vi "Starter Kit 2.0 Custom RT Host Default.vi"() -> ()   [LabVIEW 2011]
doc: "This VI shows how to use hardware abstracted sensor drivers with a custom FPGA VI to control a Starter Kit robot. This VI runs on the RT host. The main FPGA VI must be compiled before this host VI can be run."
uses:
  <vilib>/userDefined/High Color/nirio_resource_hc.ctl
  <vilib>/Platform/TimedLoop/XDataNode/timing_clust.ctl
  <vilib>/Platform/TimedLoop/XDataNode/nitl_modes.ctl
  <vilib>/Platform/TimedLoop/XDataNode/wakeup.ctl
  <instrlib>/DC Motor Controller/HAIOL/DC Motor Controller.lvclass
  <instrlib>/Hitec HS400 Series/HAIOL/Hitec HS400 Series.lvclass
  <instrlib>/Parallax PING)))/HAIOL/Parallax PING))).lvclass
  <vilib>/robotics/Utilities/RPM to Radians per Second (Scalar).vi
  <vilib>/robotics/Utilities/Radians per Second to RPM (Scalar).vi
  <vilib>/FPGAPlugInAG/sbRIO-9632/niLvFpga_Open_sbRIO-9632.vi
  <vilib>/rvi/interface/common/dynamic/niFpgaDynamicAddResources.vi
  <vilib>/Utility/AngleManip/Degrees to Radians (Scalar DBL).vi
  <vilib>/Utility/error.llb/Error Cluster From Error Code.vi
  <vilib>/rvi/errors/niLvFpgaAdjustHostInterfaceError.vi
  <vilib>/FPGAPlugInAG/Dynamic/niLvFpga_Close_Dynamic.vi
  <vilib>/Platform/TimedLoop/XDataNode/XDataNode.xnode
  <vilib>/rvi/interface/nirviOpenFPGA/nirviOpenFPGA.xnode
  FPGA Bitfiles/MintaDaNIrobotho_FPGATarget_StarterKit2.0Cus_A15A34EB.lvbitx
  Starter Kit 2.0 Custom FPGA Main.vi
  <vilib>/rvi/interface/nirviReadWriteControl/nirviReadWriteControl.xnode
  <vilib>/rvi/interface/nirviCloseFPGA/nirviCloseFPGA.xnode
  <instrlib>/DC Motor Controller/HAIOL/FPGA/DC Motor Controller FPGA.lvclass
  <instrlib>/Hitec HS400 Series/HAIOL/FPGA/Hitec HS400 Series FPGA.lvclass
  <instrlib>/Parallax PING)))/HAIOL/FPGA/Parallax PING))) FPGA.lvclass
  <vilib>/robotics/Utilities/NI_Robotics Utilities.lvlib
  <vilib>/Utility/AngleManip/NI_AngleManipulation.lvlib
  <vilib>/rvi/interface/Simulation/niFpgaSimulationCallBeginRW.vi
  NiFpgaLv.dll
  <vilib>/Platform/TimedLoop/XDataNode/XDNodeRunTimeDep.lvlib
panel:
  out "CMPS03 angle":sgl(knob) scale=0.0..360.0 scale format="%#_4f"
  in  "stop":bool
  in  "Left":dbl(slide) min=-100.0 max=100.0 step=4.0 scale=-100.0..100.0
  in  "Right":dbl(slide) min=-100.0 max=100.0 step=4.0 scale=-100.0..100.0
  out "ccw motor velocities":cluster{"Left":dbl, dbl, "Right":dbl, dbl}(graph)
  in  "sensor motor angle":dbl(slide) caption="Sensor Motor Angle (degrees)" scale=90.0..-90.0
  out "PING))) Sensor Distance (m)":dbl(graph)
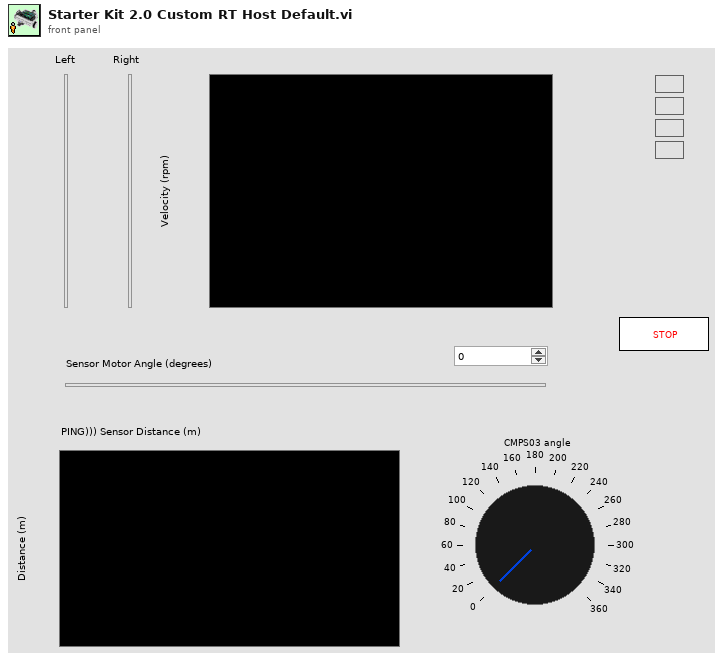
[diagram p1: front panel]
types:
  T1 = typedef "nirio_resource_hc.ctl" = tag
  T2 = typedef "XDNodeRunTimeDep.lvlib/timing_clust.ctl" = cluster{"Expected End [f-1]":u64, "Actual End [f-1]":u64, "Finished Late? [f-1]":bool, "Expected End [i-1]":u64, "Actual End [i-1]":u64, "Finished Late? [i-1]":bool, "Expected Start [i]":u64, "Actual Start [i]":u64, "Expected Start [f]":u64, "Actual Start [f]":u64, "Source Name":string, "Structure Name":string, "Period":i64, "Deadline":i64, "Offset":i64, "Start":i64, "Priority":i32, "Timeout":i32, "Mode":T3, "Wakeup Reason":T4, "Error":errorcluster, "Source Type":string, "Secondary Source Type":string, "Global End Time":u64, "Global Start Time":u64, "Frame Duration":u64, "Iteration Duration":u64, "Assigned CPU":i32, "I/O Scan Engine Mode":u32}
  T3 = typedef "XDNodeRunTimeDep.lvlib/nitl_modes.ctl" = enum32{"No Change", "Process missed periods, maintain original phase", "Discard missed periods, maintain original phase", "Process missed periods, ignore original phase", "Discard missed periods, ignore original phase"}
  T4 = typedef "XDNodeRunTimeDep.lvlib/wakeup.ctl" = enum32{"Normal", "Aborted", "Asynchronous wakeup", "Timing source error", "Timed loop error", "Timeout"}
  T5 = cluster{"Left":dbl, "rpm":dbl, "Right":dbl, "rpm":dbl}
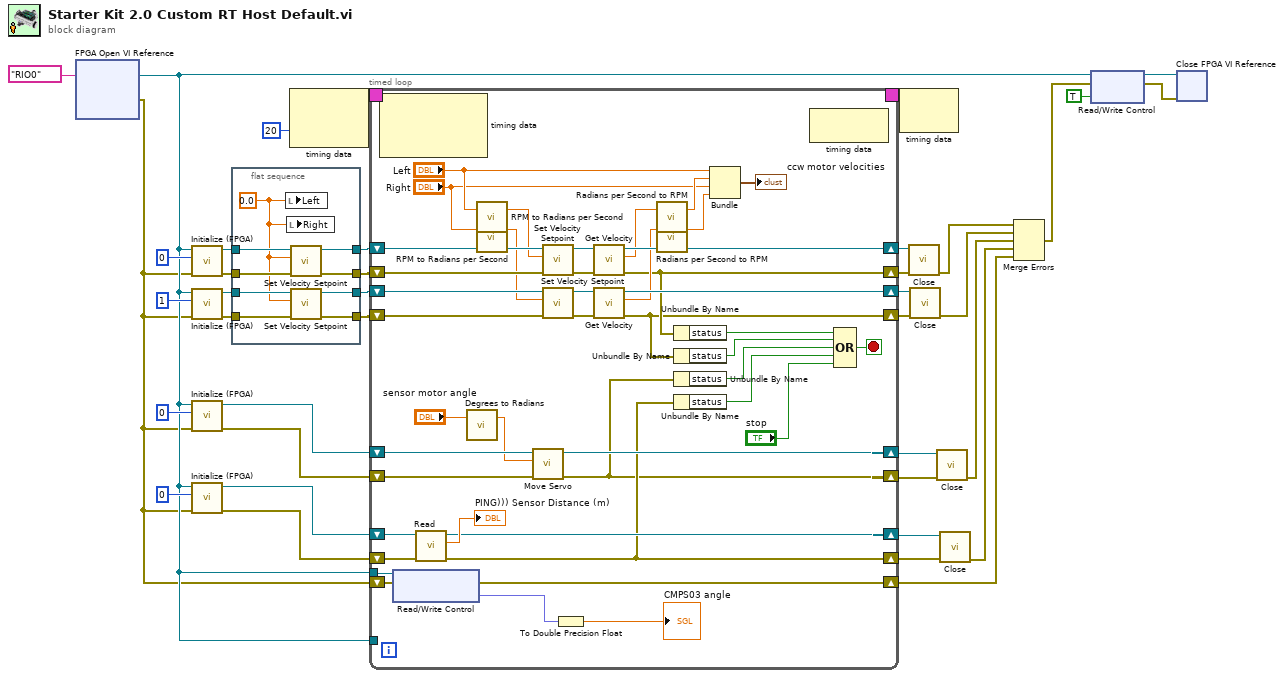
[diagram p0: block diagram]
diagram:
  n1 = xnode "FPGA Open VI Reference"("resource name"=T1 "RIO0") -> ("FPGA VI Reference Out"=w5:refnum<k20>, "error out"=w4:errorcluster)  [unwired: 1 in]
  n2 = call <instrlib>:"Initialize (FPGA).vi"("error in (no error)"=w4, "Actuator ID (0)"=0, "FPGA VI Reference"=w5) -> ("error out"=w13:errorcluster, "DC Motor Controller out"=w15:refnum<class "DC Motor Controller.lvclass">)  [unwired: 7 in]
  n3 = call <instrlib>:"Initialize (FPGA).vi"("error in (no error)"=w4, "Actuator ID (0)"=1, "FPGA VI Reference"=w5) -> ("error out"=w9:errorcluster, "DC Motor Controller out"=w11:refnum<class "DC Motor Controller.lvclass">)  [unwired: 7 in]
  n4 = call <instrlib>:"Initialize (FPGA).vi"("error in (no error)"=w4, "Actuator ID (0)"=0, "FPGA VI Reference"=w5) -> ("error out"=w25:errorcluster, "Hitec HS400 Series out"=w36:refnum<class "Hitec HS400 Series.lvclass">)  [unwired: 7 in]
  n5 = call <instrlib>:"Initialize (FPGA).vi"("error in (no error)"=w4, "Sensor ID (0)"=0, "FPGA VI Reference"=w5) -> ("error out"=w24:errorcluster, "Parallax PING))) out"=w37:refnum<class "Parallax PING))).lvclass">)  [unwired: 7 in]
  n6 = flat-sequence {
    tunnel: w15 -> [w48]
    tunnel: [w47] -> w14
    tunnel: w13 -> [w46]
    tunnel: [w45] -> w12
    tunnel: w11 -> [w44]
    tunnel: [w43] -> w10
    tunnel: w9 -> [w42]
    tunnel: [w41] -> w8
    frame #0 {
      w40 = 0.0 ("CCW Velocity (0 rad/s)")
      n7 = local write "Left"(w40) -> ()
      n8 = local write "Right"(w40) -> ()
      n9 = call-dynamic "Set Velocity Setpoint.vi"("error in (no error)"=w46, "CCW Velocity (0 rad/s)"=w40, "DC Motor Controller in"=w48) -> ("error out"=w45:errorcluster, "DC Motor Controller out"=w47:refnum<class "DC Motor Controller.lvclass">)  [unwired: 7 in]
      n10 = call-dynamic "Set Velocity Setpoint.vi"("error in (no error)"=w42, "CCW Velocity (0 rad/s)"=w40, "DC Motor Controller in"=w44) -> ("error out"=w41:errorcluster, "DC Motor Controller out"=w43:refnum<class "DC Motor Controller.lvclass">)  [unwired: 7 in]
    }
  }
  n11 = node-c288(i64 20 ("Period")) -> (w3:T2)  [unwired: 1 in]
  n12 = timed-loop {
    shift-right: [w80] -> w32
    shift-left: w37 -> [w91]
    shift-right: [w77] -> w33
    shift-left: w36 -> [w90]
    shift-right: [w87] -> w35
    shift-left: w14 -> [w89]
    shift-right: [w84] -> w34
    shift-left: w10 -> [w86]
    shift-right: [w70] -> w26
    shift-left: w12 -> [w83]
    shift-right: [w69] -> w21
    shift-left: w8 -> [w76]
    shift-right: [w67] -> w23
    shift-left: w25 -> [w78]
    shift-right: [w68] -> w22
    shift-left: w24 -> [w79]
    tunnel: w5 -> [w53]
    shift-right: [w51] -> w6
    shift-left: w4 -> [w52]
    tunnel: w5 -> [_]
    timing: w3 -> [_]
    timing-out: [_] -> w2
    stop <- w62 stop-if-true
    n13 = node-c288() -> ()  [unwired: 1 in, 3 out]
    n14 = xnode "Read/Write Control"("FPGA VI Reference In"=w53, "error in"=w52) -> ("error out"=w51:errorcluster, "CMPS03 angle"=w50:fxp<+,20,16>)  [unwired: 1 out]
    n15 = call-dynamic "Read.vi"("error in (no error)"=w79, "Parallax PING))) in"=w91) -> ("error out"=w68:errorcluster, "Distance (m)"=→"PING))) Sensor Distance (m)":dbl, "Parallax PING))) out"=w80:refnum<class "Parallax PING))).lvclass">)  [unwired: 6 in, 1 out]
    n16 = call-poly <vilib>:"Degrees to Radians.vi"("angle (deg)"="sensor motor angle") -> ("angle (rad)"=w55:dbl)  [unwired: 2 in]
    n17 = call-poly <vilib>:"RPM to Radians per Second.vi"("rpm"="Left") -> ("radians per second"=w71:dbl)  [unwired: 2 in]
    n18 = call-poly <vilib>:"RPM to Radians per Second.vi"("rpm"="Right") -> ("radians per second"=w72:dbl)  [unwired: 2 in]
    n19 = call-dynamic "Move Servo.vi"("error in (no error)"=w78, "CCW Position (0.0 rad)"=w55, "Hitec HS400 Series in"=w90) -> ("error out"=w67:errorcluster, "Hitec HS400 Series out"=w77:refnum<class "Hitec HS400 Series.lvclass">)  [unwired: 7 in]
    n20 = call-dynamic "Set Velocity Setpoint.vi"("error in (no error)"=w83, "CCW Velocity (0 rad/s)"=w71, "DC Motor Controller in"=w89) -> ("error out"=w82:errorcluster, "DC Motor Controller out"=w88:refnum<class "DC Motor Controller.lvclass">)  [unwired: 7 in]
    n21 = call-dynamic "Set Velocity Setpoint.vi"("error in (no error)"=w76, "CCW Velocity (0 rad/s)"=w72, "DC Motor Controller in"=w86) -> ("error out"=w75:errorcluster, "DC Motor Controller out"=w85:refnum<class "DC Motor Controller.lvclass">)  [unwired: 7 in]
    n22 = To Double Precision Float(number=w50) -> (double precision float=→"CMPS03 angle":dbl)
    n23 = call-dynamic "Get Velocity.vi"("error in (no error)"=w82, "DC Motor Controller in"=w88) -> ("error out"=w70:errorcluster, "CCW Velocity (rad/s)"=w74:dbl, "DC Motor Controller out"=w87:refnum<class "DC Motor Controller.lvclass">)  [unwired: 7 in]
    n24 = call-dynamic "Get Velocity.vi"("error in (no error)"=w75, "DC Motor Controller in"=w85) -> ("error out"=w69:errorcluster, "CCW Velocity (rad/s)"=w73:dbl, "DC Motor Controller out"=w84:refnum<class "DC Motor Controller.lvclass">)  [unwired: 7 in]
    n25 = call-poly <vilib>:"Radians per Second to RPM.vi"("radians per second"=w74) -> ("rpm"=w60:dbl)  [unwired: 2 in]
    n26 = call-poly <vilib>:"Radians per Second to RPM.vi"("radians per second"=w73) -> ("rpm"=w58:dbl)  [unwired: 2 in]
    n27 = Unbundle By Name(w70) -> ("status"=w66:bool)
    n28 = Unbundle By Name(w69) -> ("status"=w65:bool)
    n29 = Unbundle By Name(w67) -> ("status"=w64:bool)
    n30 = Unbundle By Name(w68) -> ("status"=w63:bool)
    n31 = Bundle("Left"="Left", "rpm"=w60, "Right"="Right", "rpm"=w58) -> (→"ccw motor velocities":T5)  [unwired: 1 in]
    n32 = node-c288() -> ()  [unwired: 1 in, 1 out]
    n33 = Compound Arithmetic op=OR(w66, w65, w64, w63, "stop") -> (w62:bool)
  }
  n34 = node-c288(w2) -> ()  [unwired: 1 out]
  n35 = call-dynamic "Close.vi"("error in (no error)"=w26, "DC Motor Controller in"=w35) -> ("error out"=w20:errorcluster)  [unwired: 9 in]
  n36 = call-dynamic "Close.vi"("error in (no error)"=w21, "DC Motor Controller in"=w34) -> ("error out"=w19:errorcluster)  [unwired: 9 in]
  n37 = call-dynamic "Close.vi"("error in (no error)"=w23, "Hitec HS400 Series in"=w33) -> ("error out"=w18:errorcluster)  [unwired: 9 in]
  n38 = call-dynamic "Close.vi"("error in (no error)"=w22, "Parallax PING))) in"=w32) -> ("error out"=w17:errorcluster)  [unwired: 9 in]
  n39 = Merge Errors(w20, w19, w18, w17, w6) -> (w16:errorcluster)
  n40 = xnode "Read/Write Control"("FPGA VI Reference In"=w5, "error in"=w16, "stop"=TRUE) -> ("FPGA VI Reference Out"=w29:refnum<k20>, "error out"=w28:errorcluster)
  n41 = xnode "Close FPGA VI Reference"("FPGA VI Reference In"=w29, "error in"=w28) -> ()  [unwired: 1 out]
